vi "cluster_v6.vi"() -> ()   [LabVIEW 2009]
panel:
  in  "Nr de perioade cosinus":dbl(knob)=25.0 scale=0.0..25.0
  out "XY Graph":cluster{dbl[], dbl[]}(graph)={[0.0, 0.9318883952751529, 0.6760759269807061, -0.44140191496238734, -0.9963087041483429, -0.28141031677181455, 0.7921482684802251, 0.8561061469101431, -0.17105162235742513, -0.980202427895276, -0.5400756633003917, 0.5883828102706561, 0.9669416441304162, 0.11312390631282306, -0.8848713552289884, -0.7550894300582629, 0.33706135033109275, 0.9996241469083186, 0.38815620273629364, -0.7180206137934257, -0.9090731435662249, 0.05849692904110355, 0.9515120941181417, 0.6318157997426203, -0.4931359037311748, -0.9895810803630345, -0.22479550267019685, 0.8264941392449691, 0.8244089265171336, -0.22839351686124176, -0.9901061917811333, -0.48991885274404895, 0.6346748502239105, 0.9503692563245907, 0.05480876090518828, -0.9106060357248796, -0.7154445439435078, 0.3915580084049592, 0.9995160538381415, 0.333581124195995, -0.7575062070501191, -0.8831444771915391, 0.11679351645065934, 0.96787703239886, 0.5853918151835941, -0.5431809892849069, -0.9794643164734751, -0.1674108037471419, 0.8580094138222696, 0.7898882514213155, -0.28495320398164936, -0.9966190171490459, -0.4380841568030572, 0.6787932411142071, 0.9305420219737283, -0.0036940948107060645, -0.9332220516705999, -0.6733493868561516, 0.4447136495821149, 0.9959847951374502, 0.27786358932900607, -0.7943974755804462, -0.8541911972456282, 0.17469010673175936, 0.9809271630993023, 0.5369629672365117, -0.5913657760605258, -0.9659930606059315, -0.10945275244283528, 0.8865861579729919, 0.7526623488268204, -0.34053697679790046, -0.9997185987245045, -0.38474910013940494, 0.7205868852590319, 0.907527845847254, -0.062184298905512164, -0.9526419472132021, -0.6289481272609245, 0.4963462251968742, 0.9890424647424783, 0.221194420833613, -0.8285680733172113, -0.8223124635893204, 0.23198841430688516, 0.9906177918309023, 0.48669511613660354, -0.6375252396890918, -0.9492134494281524, -0.05111984482792849, 0.9121265014047817, 0.7128587108633014, -0.39495447072306494, -0.9993943209890526, -0.3300963458851127, 0.7599126468221358, 0.8814055474262863, -0.12046153277942634, -0.9687992126465994, -0.582392831615603, 0.5462789028135927, 0.9787128389064523, 0.16376770058489745, -0.8599009720092948, -0.7876174552447847, 0.28849220261092656, 0.9969157299049092, 0.43476042037952345, -0.6815012921751384, -0.929182950139451, 0.007388139210379406, 0.9345429729604825, 0.6706136579479476, -0.44801931546905394, -0.9956472945365556, -0.274313070053237, 0.7966358420284375, 0.8522645909608578, -0.17832620721798967, -0.9816385121955413], [1.0, 0.25881904510252074, -0.8660254037844387, -0.7071067811865477, 0.5000000000000001, 0.9659258262890682, 3.061515884555943e-16, -0.9659258262890683, -0.49999999999999983, 0.7071067811865478, 0.8660254037844383, -0.2588190451025216, -1.0, -0.25881904510252113, 0.8660254037844386, 0.7071067811865475, -0.5000000000000003, -0.9659258262890681, 8.579020740334675e-16, 0.9659258262890685, 0.49999999999999883, -0.7071067811865487, -0.8660254037844377, 0.2588190451025228, 1.0, 0.2588190451025217, -0.8660254037844383, -0.7071067811865479, 0.4999999999999998, 0.9659258262890683, -2.455988971222789e-16, -0.9659258262890684, -0.4999999999999994, 0.7071067811865482, 0.866025403784438, -0.2588190451025222, -1.0, -0.25881904510251885, 0.8660254037844397, 0.7071067811865458, -0.5000000000000023, -0.9659258262890675, 3.186009399011591e-15, 0.9659258262890692, 0.49999999999999684, -0.7071067811865503, -0.8660254037844366, 0.258819045102525, 1.0, 0.2588190451025229, -0.8660254037844377, -0.7071067811865487, 0.4999999999999987, 0.9659258262890686, 9.790074567000984e-16, -0.9659258262890681, -0.5000000000000004, 0.7071067811865474, 0.8660254037844386, -0.258819045102521, -1.0, -0.2588190451025201, 0.8660254037844392, 0.7071067811865467, -0.5000000000000012, -0.9659258262890679, 1.961403045189214e-15, 0.9659258262890689, 0.4999999999999979, -0.7071067811865495, -0.8660254037844372, 0.25881904510252385, 1.0, 0.2588190451025172, -0.8660254037844406, -0.7071067811865446, 0.5000000000000038, 0.9659258262890671, -4.901813547078526e-15, -0.9659258262890696, -0.49999999999999534, 0.7071067811865515, 0.8660254037844357, -0.2588190451025267, -1.0, -0.25881904510251436, 0.866025403784442, 0.7071067811865425, -0.5000000000000063, -0.9659258262890663, 7.842224048967839e-15, 0.9659258262890704, 0.4999999999999928, -0.7071067811865536, -0.8660254037844343, 0.2588190451025295, 1.0, 0.25881904510252524, -0.8660254037844365, -0.7071067811865405, 0.4999999999999966, 0.9659258262890655, 3.428220164344853e-15, -0.9659258262890711, -0.5000000000000026, 0.7071067811865557, 0.8660254037844398, -0.25881904510253234, -1.0, -0.2588190451025087, 0.8660254037844379, 0.7071067811865384, -0.49999999999999917, -0.9659258262890648, -4.878096624555406e-16, 0.9659258262890719, 0.5, -0.7071067811865578, -0.8660254037844384, 0.25881904510253523]}
  in  "stop":bool
  in  "Nr de perioade sinus":dbl(knob)=22.91037367589798 scale=0.0..25.0
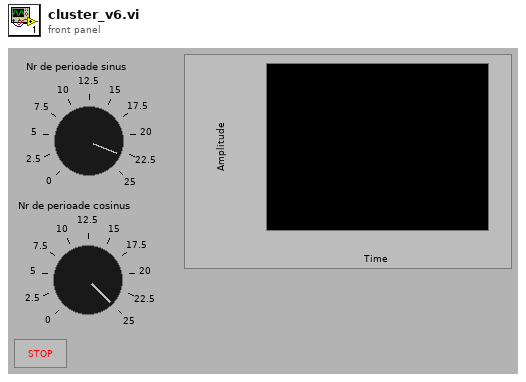
[diagram p1: front panel]
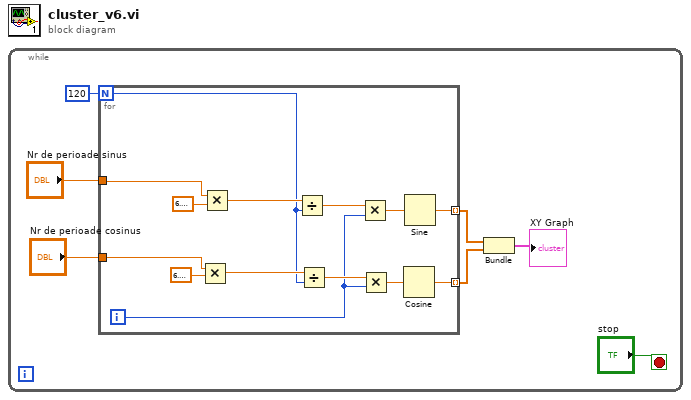
[diagram p0: block diagram]
diagram:
  n1 = while {
    stop <- "stop" stop-if-true
    n2 = for {
      N: 120 -> [w12]
      tunnel: [w21] -> w3 mode=indexing
      tunnel: "Nr de perioade sinus" -> [w17]
      tunnel: "Nr de perioade cosinus" -> [w14]
      tunnel: [w8] -> w2 mode=indexing
      i -> [w10]
      n3 = Multiply(x=w14, y=6.283185307179586) -> (x*y=w13:dbl)
      n4 = Multiply(x=w17, y=6.283185307179586) -> (x*y=w18:dbl)
      n5 = Divide(x=w18, y=w12) -> (x/y=w20:dbl)
      n6 = Divide(x=w13, y=w12) -> (x/y=w11:dbl)
      n7 = Multiply(x=w20, y=w10) -> (x*y=w19:dbl)
      n8 = Multiply(x=w11, y=w10) -> (x*y=w9:dbl)
      n9 = Cosine(x=w9) -> (cos(x)=w8:dbl)
      n10 = Sine(x=w19) -> (sin(x)=w21:dbl)
    }
    n11 = Bundle(w3, w2) -> (→"XY Graph":cluster{dbl[], dbl[]})  [unwired: 1 in]
  }
